vi "Dynamic_Switch_EOL.vi"(8 "error in (no error)":errorcluster, 9 "Value":variant[](array[variant]), 10 "Position":cluster{"Top":i16, "Left":i16}={"Top"=404, "Left"=1300}) -> (0 "error out":errorcluster, 3 "Pass/Fail":string)   [LabVIEW 2024, in "Test_2.lvlib"]
uses:
  Test_2.lvlib
  Manual_switch_EOL.vi
panel:
  out "Array 2":string[](array[string])
  out "Array":variant[](array[variant])
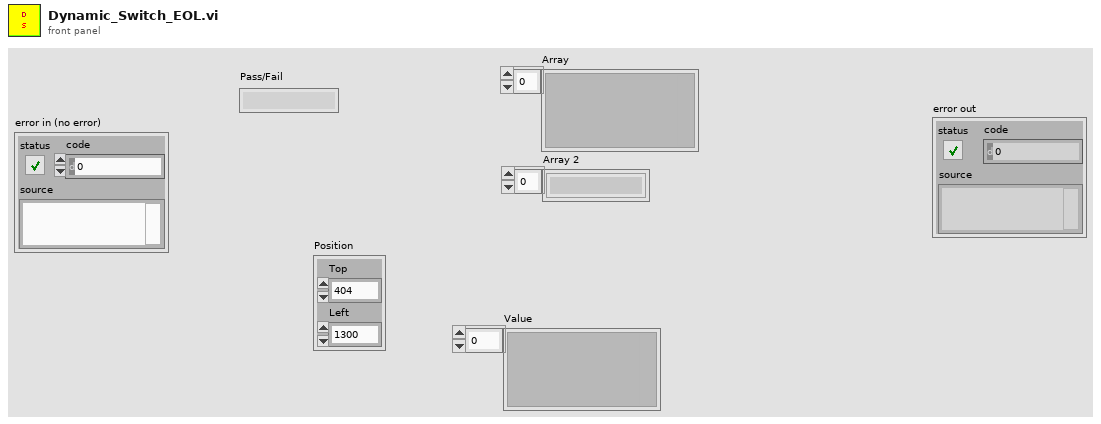
[diagram p1: front panel]
types:
  T1 = enum32{"Invalid", "Standard", "Closed", "Hidden", "Minimized", "Maximized"}
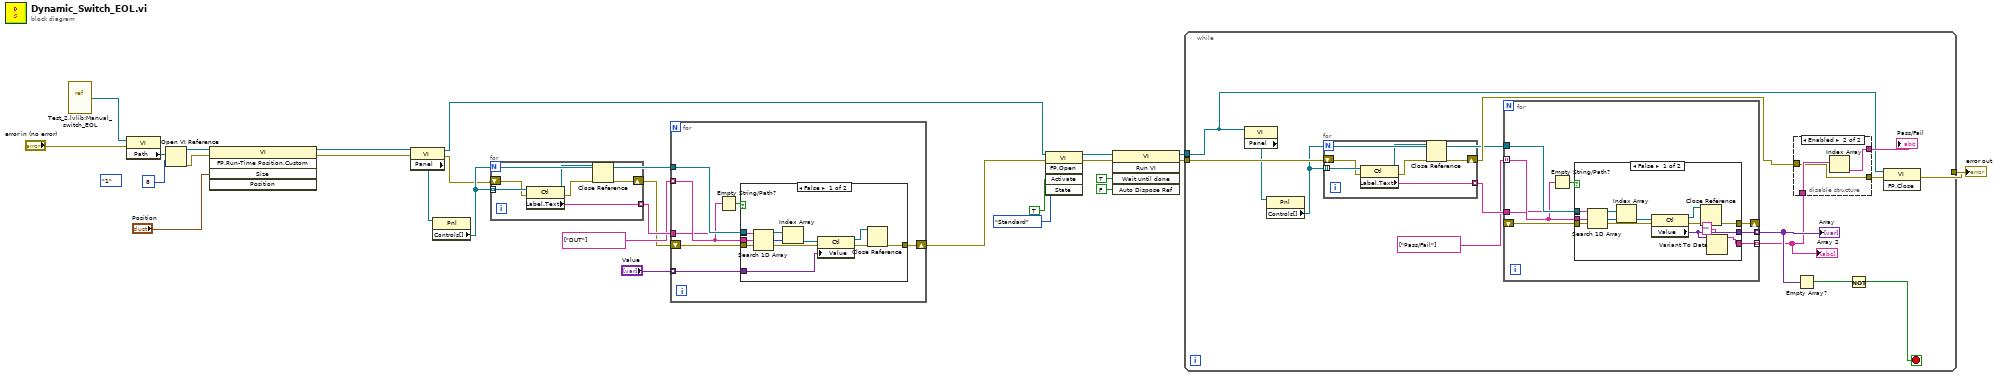
[diagram p0: block diagram]
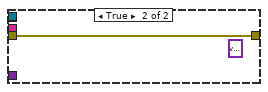
[diagram p2: hidden frame]
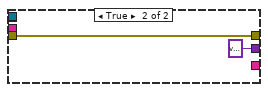
[diagram p3: hidden frame]
diagram:
  (unwired) enum16{"1", "2"}."1"
  n1 = vi-ref "Test_2.lvlib:Manual_switch_EOL.vi"() -> (w1:refnum<vi>)
  n2 = property class="VI"(reference=w1, error in="error in (no error)") -> ("Path"=w25:path)  [unwired: 2 out]
  n3 = Open VI Reference(vi path=w25, options=8) -> (vi reference=w24:refnum<vi>, error out=w14:errorcluster)  [unwired: 4 in]
  n4 = invoke class="VI" method="FP.Run-Time Position.Custom"(reference=w24, error in=w14, "Size"="Position") -> (reference out=w8:refnum<vi>, error out=w6:errorcluster)  [unwired: 2 in, 3 out]
  n5 = property class="VI"(reference=w8, error in=w6) -> (reference out=w7:refnum<vi>, error out=w5:errorcluster, "Panel"=w12:refnum<vi>)
  n6 = property class="Pnl"(reference=w12) -> ("Controls[]"=w9:refnum<vi>[])  [unwired: 1 in, 2 out]
  n7 = for {
    tunnel: w9 -> [w33] mode=indexing
    shift-right: [w29] -> w4
    shift-left: w5 -> [w32]
    tunnel: [w30] -> w11 mode=indexing
    n8 = property class="Ctl"(reference=w33, error in=w32) -> (reference out=w28:refnum<vi>, error out=w31:errorcluster, "Label.Text"=w30:string)
    n9 = Close Reference(reference=w28, error in (no error)=w31) -> (error out=w29:errorcluster)
  }
  n10 = for {
    tunnel: string[] ["DUT"] -> [w36] mode=indexing
    tunnel: w9 -> [w40]
    shift-right: [w38] -> w3
    shift-left: w4 -> [w39]
    tunnel: w11 -> [w35]
    tunnel: "Value" -> [w34] mode=indexing
    n11 = Empty String/Path?(string/path=w36) -> (empty?=w37:bool)
    n12 = case shown="False" w37 {
      tunnel: w35 -> [w50 _]
      tunnel: w36 -> [w49 _]
      tunnel: w40 -> [w48 _]
      tunnel: w39 -> [w47 w51]
      tunnel: [w43 w51] -> w38
      tunnel: w34 -> [w41 _]
      frame False {
        n13 = Search 1D Array(1D array=w50, element=w49) -> (index of element=w46:i32)  [unwired: 1 in]
        n14 = Index Array(array=w48, index=w46) -> (element=w45:refnum<vi>)
        n15 = property class="Ctl"(reference=w45, error in=w47, "Value"=w41) -> (reference out=w42:refnum<vi>, error out=w44:errorcluster)
        n16 = Close Reference(reference=w42, error in (no error)=w44) -> (error out=w43:errorcluster)
      }
      frame True {
        (unwired) variant ("Value")
      }
    }
  }
  n17 = invoke class="VI" method="FP.Open"(reference=w7, error in=w3, "Activate"=TRUE ("Activate?"), "State"=T1."Standard") -> (reference out=w17:refnum<vi>, error out=w16:errorcluster)  [unwired: 1 in, 3 out]
  n18 = invoke class="VI" method="Run VI"(reference=w17, error in=w16, "Wait until done"=TRUE ("Wait Until Done"), "Auto Dispose Ref"=FALSE ("Auto Dispose Reference")) -> (reference out=w26:refnum<vi>, error out=w27:errorcluster)  [unwired: 1 in, 3 out]
  n19 = while {
    tunnel: w27 -> [w64]
    tunnel: w26 -> [w52]
    tunnel: [w53] -> w13
    stop <- w56 stop-if-true
    n20 = property class="VI"(reference=w52) -> ("Panel"=w63:refnum<vi>)  [unwired: 1 in, 2 out]
    n21 = property class="Pnl"(reference=w63) -> ("Controls[]"=w59:refnum<vi>[])  [unwired: 1 in, 2 out]
    n22 = for {
      tunnel: w59 -> [w71] mode=indexing
      shift-right: [w67] -> w62
      shift-left: w64 -> [w70]
      tunnel: [w68] -> w61 mode=indexing
      n23 = property class="Ctl"(reference=w71, error in=w70) -> (reference out=w66:refnum<vi>, error out=w69:errorcluster, "Label.Text"=w68:string)
      n24 = Close Reference(reference=w66, error in (no error)=w69) -> (error out=w67:errorcluster)
    }
    n25 = for {
      tunnel: string[] ["Pass/Fail"] -> [w75] mode=indexing
      tunnel: w59 -> [w79]
      shift-right: [w77] -> _
      shift-left: _ -> [w78]
      tunnel: [w74] -> w58 mode=indexing
      tunnel: w61 -> [w73]
      tunnel: [w72] -> w55 mode=indexing
      n26 = Empty String/Path?(string/path=w75) -> (empty?=w76:bool)
      n27 = case shown="False" w76 {
        tunnel: w73 -> [w91 _]
        tunnel: w75 -> [w90 _]
        tunnel: w79 -> [w89 _]
        tunnel: w78 -> [w88 w93]
        tunnel: [w84 w93] -> w77
        tunnel: [w82 variant ("Value")] -> w74
        tunnel: [w80 _] -> w72
        frame False {
          n28 = Search 1D Array(1D array=w91, element=w90) -> (index of element=w87:i32)  [unwired: 1 in]
          n29 = Index Array(array=w89, index=w87) -> (element=w86:refnum<vi>)
          n30 = property class="Ctl"(reference=w86, error in=w88) -> (reference out=w83:refnum<vi>, error out=w85:errorcluster, "Value"=w82:variant)
          n31 = Close Reference(reference=w83, error in (no error)=w85) -> (error out=w84:errorcluster)
          n32 = Variant To Data(type="", Variant=w82) -> (data=w80:string)  [unwired: 1 in, 1 out]
        }
        frame True {
        }
      }
    }
    "Array" <- w58
    "Array 2" <- w55
    n33 = disable-structure shown="Enabled" {
      disable-tunnel: [_ w95] -> w65
      disable-tunnel: w62 -> [_ w94]
      disable-tunnel: w55 -> [_ w96]
      disable-tunnel: [_ w94] -> w54
      frame Disabled {
      }
      frame Enabled {
        n34 = Index Array(array=w96) -> (element=w95:string)  [unwired: 1 in]
      }
    }
    "Pass/Fail" <- w65
    n35 = Empty Array?(array=w58) -> (empty?=w57:bool)
    n36 = Not(x=w57) -> (.not. x?=w56:bool)
    n37 = invoke class="VI" method="FP.Close"(reference=w52, error in=w54) -> (error out=w53:errorcluster)  [unwired: 1 in, 2 out]
  }
  "error out" <- w13
